vi "CtrlTreeProcessSelection.vi"(11 "Selection":string[](array[string])) -> (3 "Map":map{string, string}(c390))   [LabVIEW 2021]
uses:
  <vilib>/regexp/Match Regular Expression.xnode
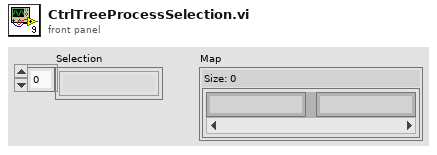
[diagram p1: front panel]
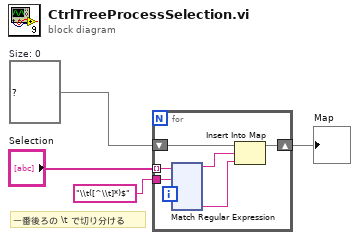
[diagram p0: block diagram]
diagram:
  w3 = map{string, string} {}  # Size: 0
  # "一番後ろの \\t で切り分ける"
  n1 = for {
    tunnel: "Selection" -> [w10] mode=indexing
    tunnel: "\\t([^\\t]*)$" ("regular expression") -> [w9]
    shift-right: [w7] -> w1
    shift-left: w3 -> [w8]
    n2 = xnode "Match Regular Expression"("input string"=w10, "regular expression"=w9) -> ("before match"=w6:string, "submatch 1"=w5:string)  [unwired: 4 in, 4 out]
    n3 = Insert Into Map(map in=w8, key=w6, value=w5) -> (map out=w7:map{string, string})  [unwired: 2 out]
  }
  "Map" <- w1
